vi "motor.vi"   [LabVIEW 2018]
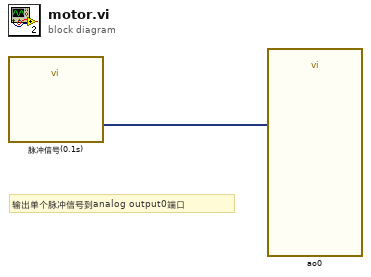
[diagram p0: block diagram]
diagram:
  # "输出单个脉冲信号到analog output0端口"
  n1 = call "脉冲信号(0.1s)"() -> ("Signal"=w1:dynamicdata)  [unwired: 9 in, 2 out]
  n2 = call "ao0"("data"=w1) -> ()  [unwired: 17 in, 2 out]
